vi "Replace Array Subset (Single).vi"(0 "JSON Array":refnum<class "JSON Value.lvclass">, 7 "index":i32, 9 "new element/subarray":refnum<class "JSON Value.lvclass">, 11 "error in":errorcluster) -> (4 "output JSON Array":refnum<class "JSON Value.lvclass">, 15 "error out":errorcluster)   [LabVIEW 2016, in "JSON Value.lvclass"]
doc: "Replaces an element or subarray in an array at the point you specify in index."
uses:
  JSON Value.lvclass
  JSON Value.lvclass/JSON Value.ctl
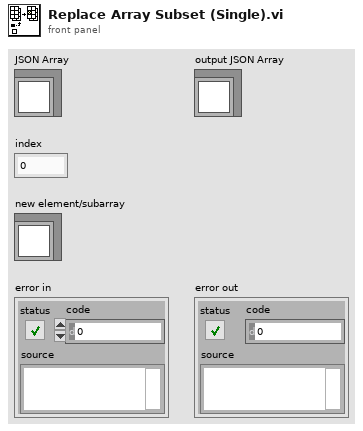
[diagram p1: front panel]
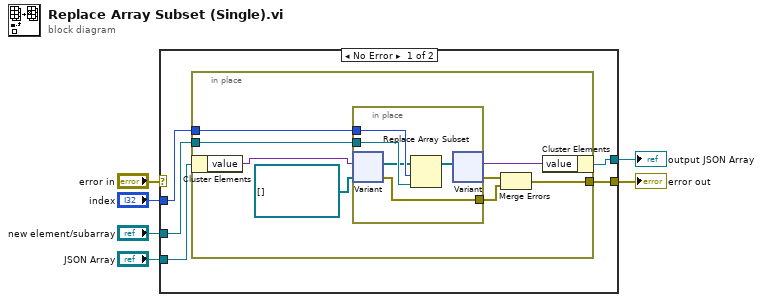
[diagram p0: block diagram]
diagram:
  n1 = case shown="No Error" "error in" {
    selector: "error in" -> [_ w26]
    tunnel: "JSON Array" -> [w11 w25]
    tunnel: "new element/subarray" -> [w10 _]
    tunnel: "index" -> [w9 _]
    tunnel: [w8 w25] -> w3
    tunnel: [w7 w26] -> w2
    frame No Error {
      n2 = in-place {
        in-place-border: w10 -> [w19]
        in-place-border: w9 -> [w18]
        in-place-border: [w12] -> w7
        n3 = in-place-cluster #1(w11) -> ("value"=w17:variant)
        n4 = in-place {
          in-place-border: w19 -> [w24]
          in-place-border: w18 -> [w23]
          in-place-border: [w20] -> w14
          n5 = in-place-variant #2(w17, refnum<class "JSON Value.lvclass">[] [] ("new element/subarray")) -> (w22:refnum<class "JSON Value.lvclass">[], w20:errorcluster)
          n6 = Replace Array Subset(array=w22, new element=w24, index=w23) -> (w21:refnum<class "JSON Value.lvclass">[])
          n7 = in-place-variant #2(w21) -> (w16:variant, w13:errorcluster)
        }
        n8 = Merge Errors(w13, w14) -> (w12:errorcluster)
        n9 = in-place-cluster #1("value"=w16) -> (w8:refnum<class "JSON Value.lvclass">)
      }
    }
    frame Error {
    }
  }
  "output JSON Array" <- w3
  "error out" <- w2
